vi "CommonVIs_UpdateClassInheritance.vi"(2 "ClassPath/LvClassRef":variant, 3 "ParentClass":path, 5 "error in (no error)":errorcluster, 7 "Don'tShowDialog(False)":bool) -> (19 "error out":errorcluster)   [LabVIEW 2020]
uses:
  Provider_BaseClassInterface/ClassReader_class/ClassReader.lvclass
  Provider_BaseClassInterface/ClassWriter_class/ClassWriter.lvclass
  Provider_LvNativeClass/ClassWriterNative_class/ClassWriterNative.lvclass
panel:
  out "Updating Inheritance":u8(slide) scale=0.0..100.0
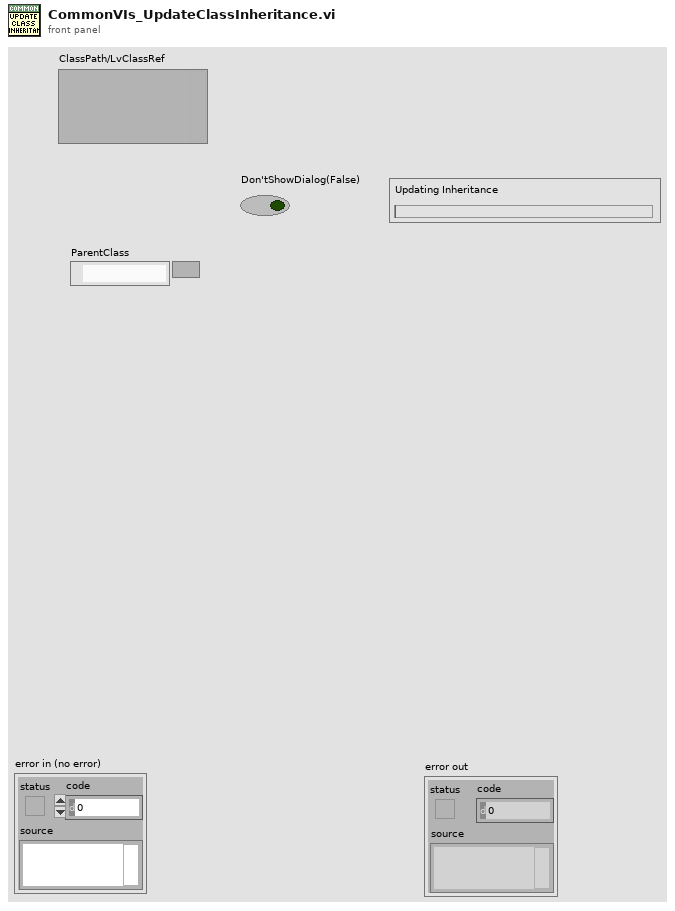
[diagram p1: front panel]
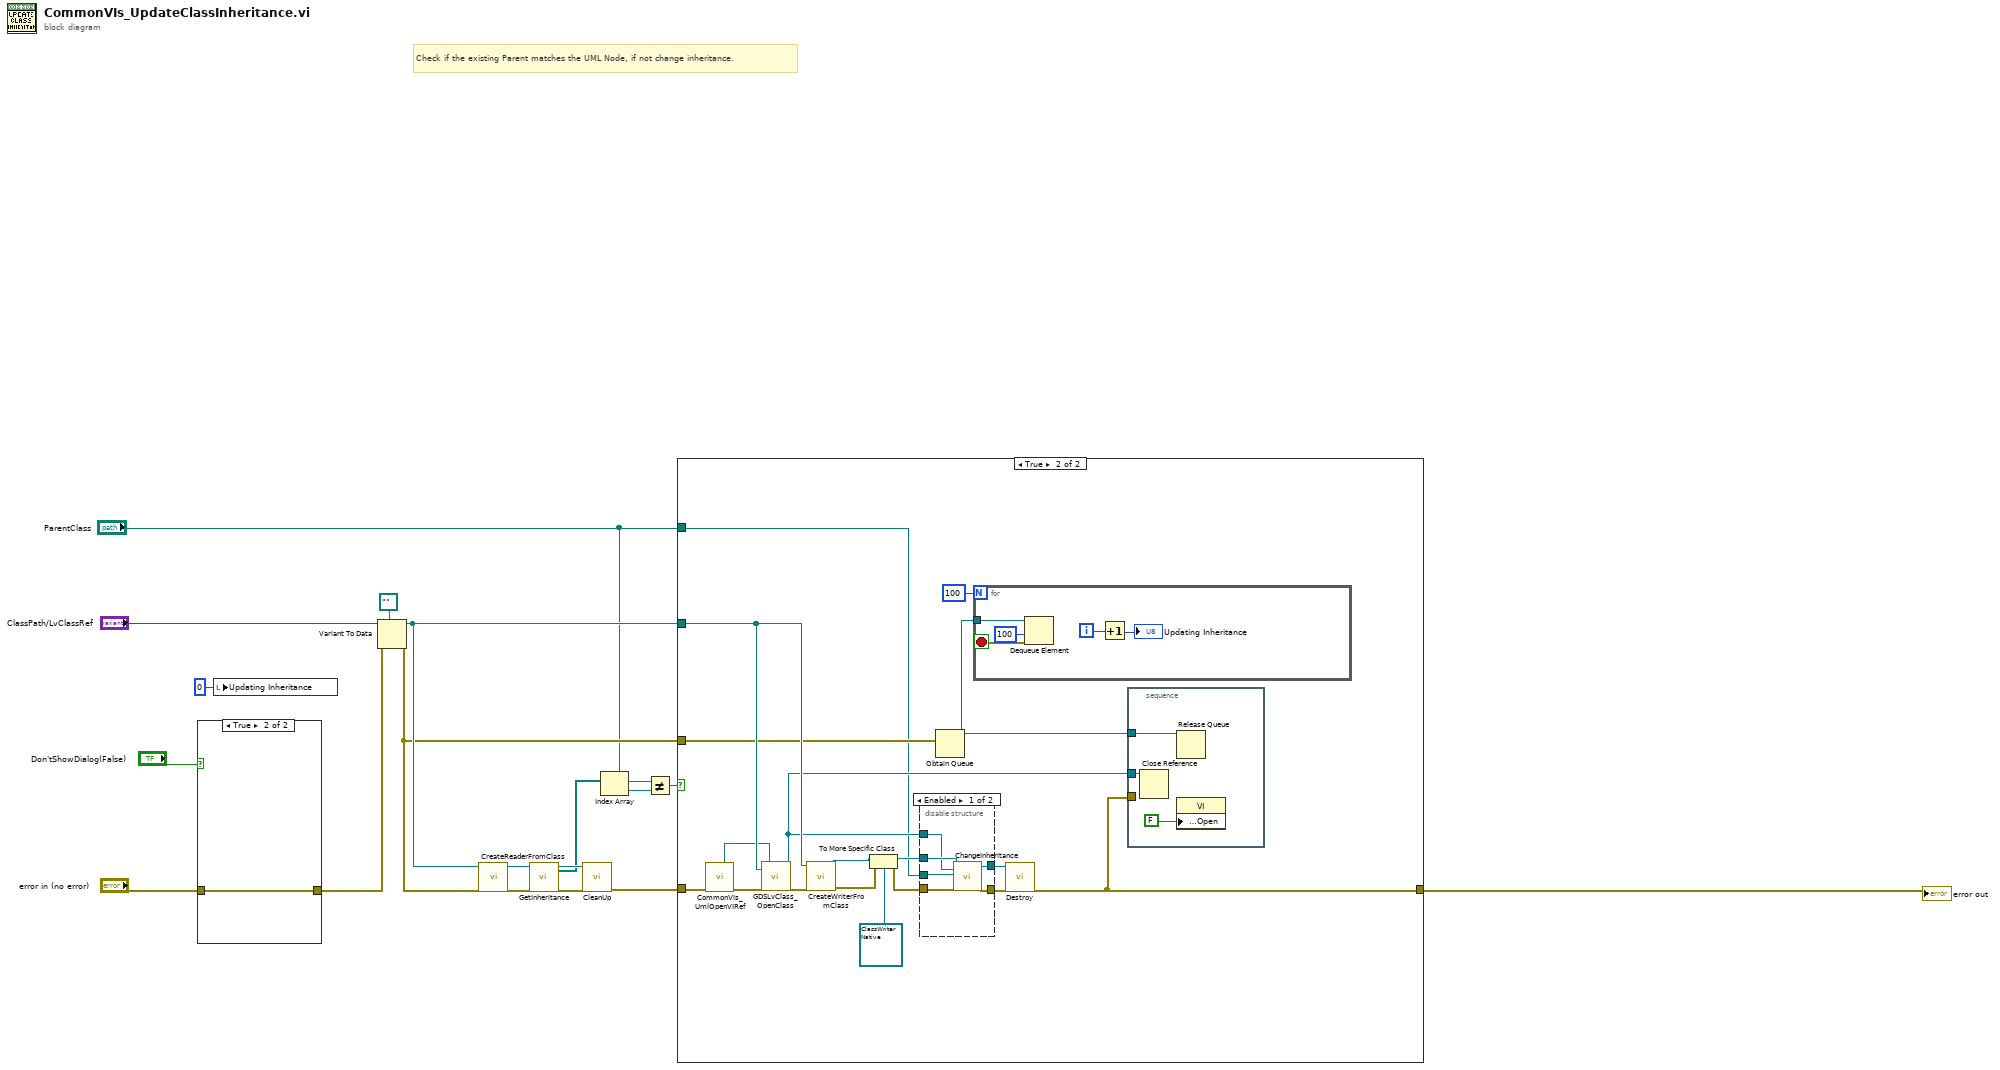
[diagram p0: block diagram]
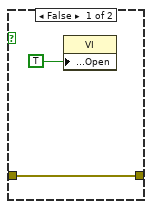
[diagram p4: hidden frame]
diagram:
  # "Check if the existing Parent matches the UML Node, if not change inheritance."
  n1 = case shown="True" "Don'tShowDialog(False)" {
    tunnel: "error in (no error)" -> [w19 w21]
    tunnel: [w19 w21] -> w7
    frame False {
      n2 = property class="VI"("Front Panel.Open"=TRUE ("Front Panel Window:Open")) -> ()  [unwired: 2 in, 2 out]
    }
    frame True {
    }
  }
  n3 = local write "Updating Inheritance"(u8 0 ("Updating Inheritance")) -> ()
  n4 = Variant To Data(error in=w7, type=path "", Variant="ClassPath/LvClassRef") -> (data=w10:path, error out=w6:errorcluster)
  n5 = call "CreateReaderFromClass.vi"("ClassPath/LvClassRef"=w10, "error in"=w6) -> ("ClassReader"=w16:refnum<class "ClassReader.lvclass">, "error out"=w15:errorcluster)  [unwired: 16 out]
  n6 = call-dynamic "GetInheritance.vi"("ClassReader in"=w16, "error in (no error)"=w15) -> ("ClassReader out"=w14:refnum<class "ClassReader.lvclass">, "Inheritance"=w4:path[], "error out"=w13:errorcluster)  [unwired: 14 in, 1 out]
  n7 = call-dynamic "CleanUp.vi"("reference in"=w14, "error in (no error)"=w13) -> ("error out"=w11:errorcluster)  [unwired: 17 out]
  n8 = Index Array(array=w4) -> (element=w3:path)  [unwired: 1 in]
  n9 = Not Equal?(x="ParentClass", y=w3) -> (x != y?=w1:bool)
  n10 = case shown="True" w1 {
    tunnel: w11 -> [w22 w34]
    tunnel: w10 -> [_ w33]
    tunnel: [w22 w28] -> w9
    tunnel: w6 -> [_ w26]
    tunnel: "ParentClass" -> [_ w23]
    frame False {
    }
    frame True {
      n11 = call "CommonVIs_UmlOpenVIRef.vi"("error in"=w34) -> ("error out"=w32:errorcluster, "AppRefOut"=w31:refnum<vi>)  [unwired: 3 in, 6 out]
      n12 = call "GDSLvClass_OpenClass.vi"("ClassToOpen"=w33, "error in (no error)"=w32, "Project/ApplicationRef(If empty, currect active project will be used)"=w31) -> ("LVClass.Open"=w24:refnum<vi>, "error out"=w35:errorcluster)  [unwired: 15 out]
      n13 = call "CreateWriterFromClass.vi"("ClassPath/LvClassRef"=w33, "error in"=w35) -> ("ClassWriter"=w40:refnum<class "ClassWriter.lvclass">, "error out"=w39:errorcluster)  [unwired: 16 out]
      n14 = To More Specific Class(target class=refnum<class "ClassWriterNative.lvclass"> refnum ("reference in"), reference=w40, error in=w39) -> (specific class reference=w37:refnum<class "ClassWriterNative.lvclass">, error out=w36:errorcluster)
      n15 = disable-structure shown="Enabled" {
        disable-tunnel: w37 -> [w51 w52]
        disable-tunnel: w36 -> [w50 w53]
        disable-tunnel: w24 -> [w49 _]
        disable-tunnel: [w48 w52] -> w30
        disable-tunnel: [w47 w53] -> w29
        disable-tunnel: w23 -> [w46 _]
        frame Enabled {
          n16 = call-dynamic "ChangeInheritance.vi"("ClassWriterGOOP300 in"=w51, "LvClass"=w49, "NewBaseClass(Empty=ConvertClassToBaseClass)"=w46, "error in (no error)"=w50) -> ("ClassWriterGOOP300 out"=w48:refnum<class "ClassWriterNative.lvclass">, "error out"=w47:errorcluster)  [unwired: 14 in]
        }
        frame Disabled {
        }
      }
      n17 = Obtain Queue(element data type=w26) -> (queue out=w25:refnum<queue>)  [unwired: 4 in, 2 out]
      n18 = for {
        N: 100 -> [_]
        tunnel: w25 -> [w44]
        i -> [w42]
        stop <- w43 stop-if-true
        n19 = Dequeue Element(queue=w44, timeout in ms (-1)=100) -> (error out=w43:errorcluster)  [unwired: 1 in, 3 out]
        n20 = Increment(x=w42) -> (x+1=→"Updating Inheritance":i32)
      }
      n21 = call-dynamic "Destroy.vi"("ClassWriterNative"=w30, "error in (no error)"=w29) -> ("error out"=w28:errorcluster)  [unwired: 17 out]
      n22 = stacked-sequence {
        tunnel: w28 -> [_]
        tunnel: w25 -> [w55]
        tunnel: w24 -> [w54]
        frame #0 {
          n23 = Close Reference(reference=w54) -> ()  [unwired: 1 in, 1 out]
          n24 = Release Queue(queue=w55) -> ()  [unwired: 2 in, 3 out]
          n25 = property class="VI"("Front Panel.Open"=FALSE ("Front Panel Window:Open")) -> ()  [unwired: 2 in, 2 out]
        }
      }
    }
  }
  "error out" <- w9
